vi "Test of Calibration interface.vi"   [LabVIEW 2020, in "PathControl.lvclass"]
uses:
  PathControl.lvclass
  Instruments/Vector Network Analyzer/VNA-ZNB/VNA-ZNB.lvclass
  C:/Sandbox/RF Bench/Source Code/WiSpry Test Framework/Instruments/Instrument.lvclass
  C:/Sandbox/RF Bench/Source Code/WiSpry Test Framework/Instruments/Vector Network Analyzer/Vector Network Analyzer.lvclass
  Instruments/Instrument.lvclass/Instrument.ctl
  PathControl.lvclass/PathControl.ctl
  Instruments/Instrument.lvclass
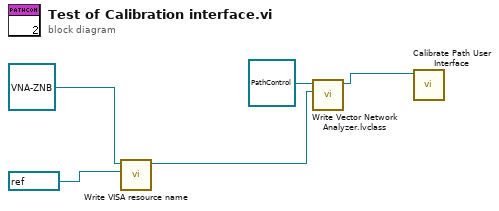
[diagram p0: block diagram]
diagram:
  n1 = call "Write VISA resource name.vi"("VISA resource name"=refnum<visa-resource-name> "ZNB", "Instrument in"=refnum<class "VNA-ZNB.lvclass"> refnum ("VNA-ZNB.lvclass")) -> ("Instrument out"=w1:refnum<class "VNA-ZNB.lvclass">)  [unwired: 9 in]
  n2 = call "Write Vector Network Analyzer.lvclass.vi"("Vector Network Analyzer.lvclass"=w1, "PathControl in"=refnum<class "PathControl.lvclass"> refnum) -> ("PathControl out"=w3:refnum<class "PathControl.lvclass">)  [unwired: 9 in]
  n3 = call "Calibrate Path User Interface.vi"("PathControl in"=w3) -> ()  [unwired: 9 in, 2 out]
